vi "FGVFINAL.vi"() -> ()   [LabVIEW 2013]
panel:
  out "FINAL POSITION":dbl
  out "LOOP SUM":i32
  in  "stop":bool
  in  "initial position":i32
  # "press again after stop is pressed initally"
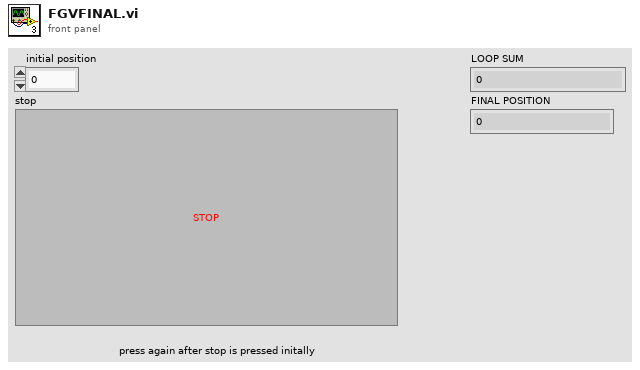
[diagram p1: front panel]
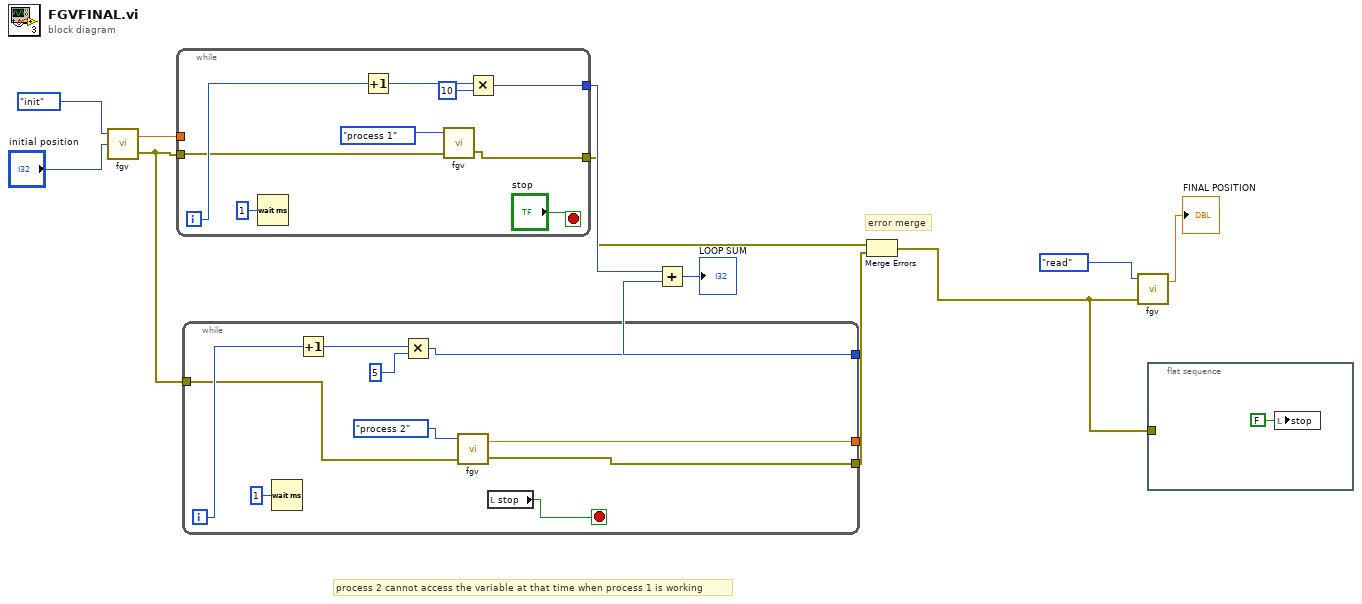
[diagram p0: block diagram]
diagram:
  # "process 2 cannot access the variable at that time when process 1 is working"
  # "error merge"
  n1 = call "fgv.vi"("initial position"="initial position", "Enum"=enum16{"init", "process 1", "process 2", "read"}."init") -> ("error out"=w6:errorcluster, "new position"=w7:dbl)  [unwired: 1 in]
  n2 = while {
    tunnel: [w16] -> w12
    tunnel: w7 -> [_]
    tunnel: w6 -> [w14]
    tunnel: [w13] -> w3
    i -> [w17]
    stop <- "stop" stop-if-true
    n3 = Wait (ms)(milliseconds to wait=u32 1) -> ()  [unwired: 1 out]
    n4 = Increment(x=w17) -> (x+1=w19:i32)
    n5 = call "fgv.vi"("error in (no error)"=w14, "Enum"=enum16{"init", "process 1", "process 2", "read"}."process 1") -> ("error out"=w13:errorcluster)  [unwired: 1 in, 1 out]
    n6 = Multiply(x=w19, y=10) -> (x*y=w16:i32)
  }
  n7 = while {
    tunnel: [w26] -> w11
    tunnel: w6 -> [w24]
    tunnel: [w23] -> w2
    tunnel: [w22] -> _
    i -> [w27]
    stop <- w31 stop-if-true
    n8 = Wait (ms)(milliseconds to wait=u32 1) -> ()  [unwired: 1 out]
    n9 = Increment(x=w27) -> (x+1=w29:i32)
    n10 = Multiply(x=w29, y=5) -> (x*y=w26:i32)
    n11 = call "fgv.vi"("error in (no error)"=w24, "Enum"=enum16{"init", "process 1", "process 2", "read"}."process 2") -> ("error out"=w23:errorcluster, "new position"=w22:dbl)  [unwired: 1 in]
    n12 = local read "stop"() -> (w31:bool)
  }
  n13 = Add(x=w12, y=w11) -> (x+y=→"LOOP SUM":i32)
  n14 = Merge Errors(w3, w2) -> (w1:errorcluster)
  n15 = call "fgv.vi"("error in (no error)"=w1, "Enum"=enum16{"init", "process 1", "process 2", "read"}."read") -> ("new position"=→"FINAL POSITION":dbl)  [unwired: 1 in, 1 out]
  n16 = flat-sequence {
    tunnel: w1 -> [_]
    frame #0 {
      n17 = local write "stop"(FALSE ("stop")) -> ()
    }
  }
